vi "Result.Numeric Look Up Limits.vi"(0 "Measurement":T1 {"Status" items=["LOG", "PASS", "FAIL", "ERROR"]}, 4 "Limits":variant) -> (5 "Measurement Out":T1 {"Status" items=["LOG", "PASS", "FAIL", "ERROR"]})   [LabVIEW 2018]
uses:
  Result.Numeric.ctl
  Result.Limit Type.ctl
  Result.Measurement and Attribute Item Status.ctl
  Result.Test Limit Item.ctl
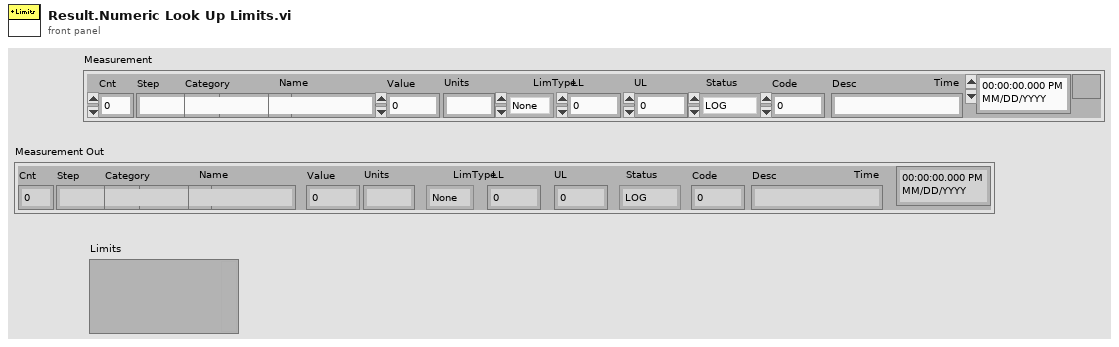
[diagram p1: front panel]
types:
  T1 = typedef "Result.Numeric.ctl" = cluster{"Cnt":i32, "Step":string, "Category":string, "Name":string, "Value":dbl, "Units":string, "LimType":T2, "LL":dbl, "UL":dbl, "Status":T3, "Code":i32, "Desc":string, "Time":timestamp}
  T2 = typedef "Result.Limit Type.ctl" = enum16{"None", "EQ", "NE", "GT", "LT", "GE", "LE", "GTLT", "GELE", "GELT", "GTLE", "LTGT", "LEGE", "LEGT", "LTGE", "Contains", "NotContains"}
  T3 = typedef "Result.Measurement and Attribute Item Status.ctl" = i32
  T4 = typedef "Result.Test Limit Item.ctl" = cluster{"Name":string, "LimType":T2, "LL":string, "UL":string, "Units":string, "FailCode":i32, "FailDesc":string}
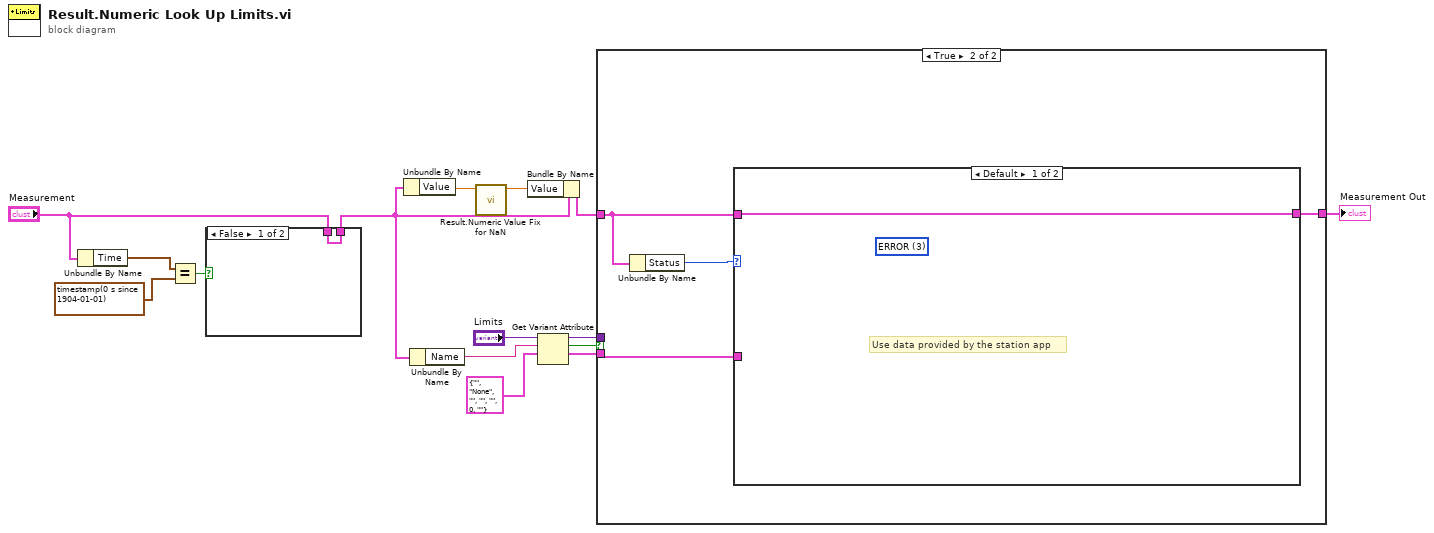
[diagram p0: block diagram]
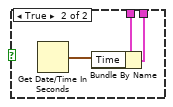
[diagram p2: hidden frame]
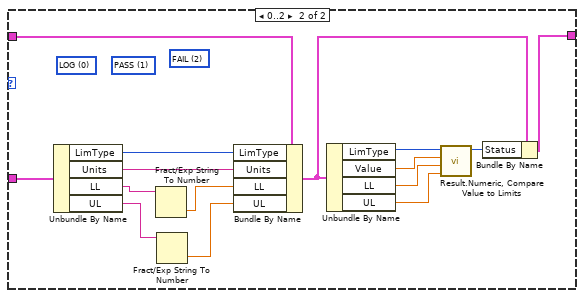
[diagram p4: hidden frame]
diagram:
  n1 = Unbundle By Name("Measurement") -> ("Time"=w7:timestamp)
  n2 = Equal?(x=w7, y=timestamp(0 s since 1904-01-01) ("Time")) -> (x = y?=w5:bool)
  n3 = case shown="False" w5 {
    tunnel: [w16 w19] -> w2
    tunnel: "Measurement" -> [w16 w17]
    frame False {
    }
    frame True {
      n4 = Get Date/Time In Seconds() -> (seconds since 1Jan1904=w18:timestamp)
      n5 = Bundle By Name(cluster=w17, "Time"=w18) -> (w19:T1)
    }
  }
  n6 = Unbundle By Name(w2) -> ("Value"=w3:dbl)
  n7 = Unbundle By Name(w2) -> ("Name"=w14:string)
  n8 = call "Result.Numeric Value Fix for NaN.vi"("Numeric"=w3) -> ("Numeric Out"=w4:dbl)  [unwired: 10 in]
  n9 = Bundle By Name(cluster=w2, "Value"=w4) -> (w1:T1)
  n10 = Get Variant Attribute(Variant="Limits", name=w14, default value (empty Variant)=T4 {"Name"="", "LimType"=enum."None", "LL"="", "UL"="", "Units"="", "FailCode"=0, "FailDesc"=""} ("Result.Test Limit Item")) -> (duplicate Variant=w11:variant, found=w12:bool, value=w10:T4)  [unwired: 1 in, 1 out]
  n11 = case shown="True" w12 {
    tunnel: w11 -> [_ _]
    tunnel: w10 -> [_ w24]
    tunnel: w1 -> [w20 w22]
    tunnel: [w20 w23] -> w9
    frame False {
      # "If not found use data provided by the station app"
    }
    frame True {
      n12 = Unbundle By Name(w22) -> ("Status"=w21:T3)
      n13 = case shown="Default" w21 {
        tunnel: w24 -> [_ w39]
        tunnel: [w25 w38] -> w23
        tunnel: w22 -> [w25 w31]
        frame Default {
          (unwired) T3 3 items=["LOG", "PASS", "FAIL", "ERROR"] ("y")
          # "Use data provided by the station app"
        }
        frame 0..2 {
          (unwired) T3 2 items=["LOG", "PASS", "FAIL", "ERROR"] ("y")
          (unwired) T3 1 items=["LOG", "PASS", "FAIL", "ERROR"] ("y")
          (unwired) T3 0 items=["LOG", "PASS", "FAIL", "ERROR"] ("y")
          n14 = Unbundle By Name(w39) -> ("LimType"=w40:T2, "Units"=w36:string, "LL"=w35:string, "UL"=w34:string)
          n15 = Fract/Exp String To Number(string=w35) -> (number=w33:dbl)  [unwired: 3 in, 1 out]
          n16 = Fract/Exp String To Number(string=w34) -> (number=w32:dbl)  [unwired: 3 in, 1 out]
          n17 = Bundle By Name(cluster=w31, "LimType"=w40, "Units"=w36, "LL"=w33, "UL"=w32) -> (w37:T1)
          n18 = Unbundle By Name(w37) -> ("LimType"=w29:T2, "Value"=w28:dbl, "LL"=w27:dbl, "UL"=w26:dbl)
          n19 = call "Result.Numeric, Compare Value to Limits.vi"("UL"=w26, "LL"=w27, "Value"=w28, "LimType"=w29) -> ("Status"=w30:T3)  [unwired: 7 in]
          n20 = Bundle By Name(cluster=w37, "Status"=w30) -> (w38:T1)
        }
      }
    }
  }
  "Measurement Out" <- w9
